vi "DROPBEAR_Model_Updating_FFT.vi"(8 "error in (no error)":errorcluster, 11 "DROPBEAR_Model_Updating in":refnum<class "DROPBEAR_Model_Updating.lvclass">=refnum) -> (0 "error out":errorcluster, 3 "DROPBEAR_Model_Updating out":refnum<class "DROPBEAR_Model_Updating.lvclass">, 4 "looping":bool=TRUE)   [LabVIEW 2021, in "DROPBEAR_Model_Updating.lvclass"]
uses:
  DROPBEAR_Model_Updating.lvclass
  MOCKBEAR/MOCKBEAR.lvclass
  FEA_Model/FEA_Model.lvclass
  Kalman_Filter/Kalman_Filter.lvclass
  Data_Array/Data_Array.lvclass
  Moving_Statistic/Moving_Statistic.lvclass
  Online_Statistic/Online_Statistic.lvclass
  <vilib>/Analysis/4window.llb/Hanning Window (DBL).vi
  <vilib>/Analysis/5stat.llb/RMS (DBL).vi
  <vilib>/Analysis/2dsp.llb/Real FFT.vi
  <vilib>/Analysis/4window.llb/AllCosWindow (DBL).vi
  <vilib>/Analysis/NI_AALPro.lvlib
panel:
  in  "Bound to 1st Frequency":bool=TRUE
  in  "Frequency Method":T1(ring)=enum."FFT"
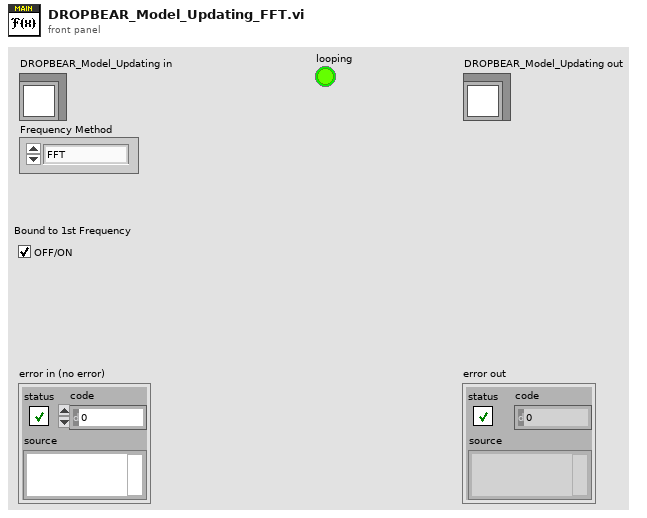
[diagram p1: front panel]
types:
  T1 = enum16{"Bandpass FFT", "Tone", "FFT", "Custom Filter"}
  T2 = cluster{"Time Cycle Start":u32, "Time Data Acquire":u32, "Time FFT":u32, "Time KF FFT":u32, "Time Sample":u32, "Time FEA":u32, "Time KF FEA":u32, "Time Cycle End":u32}
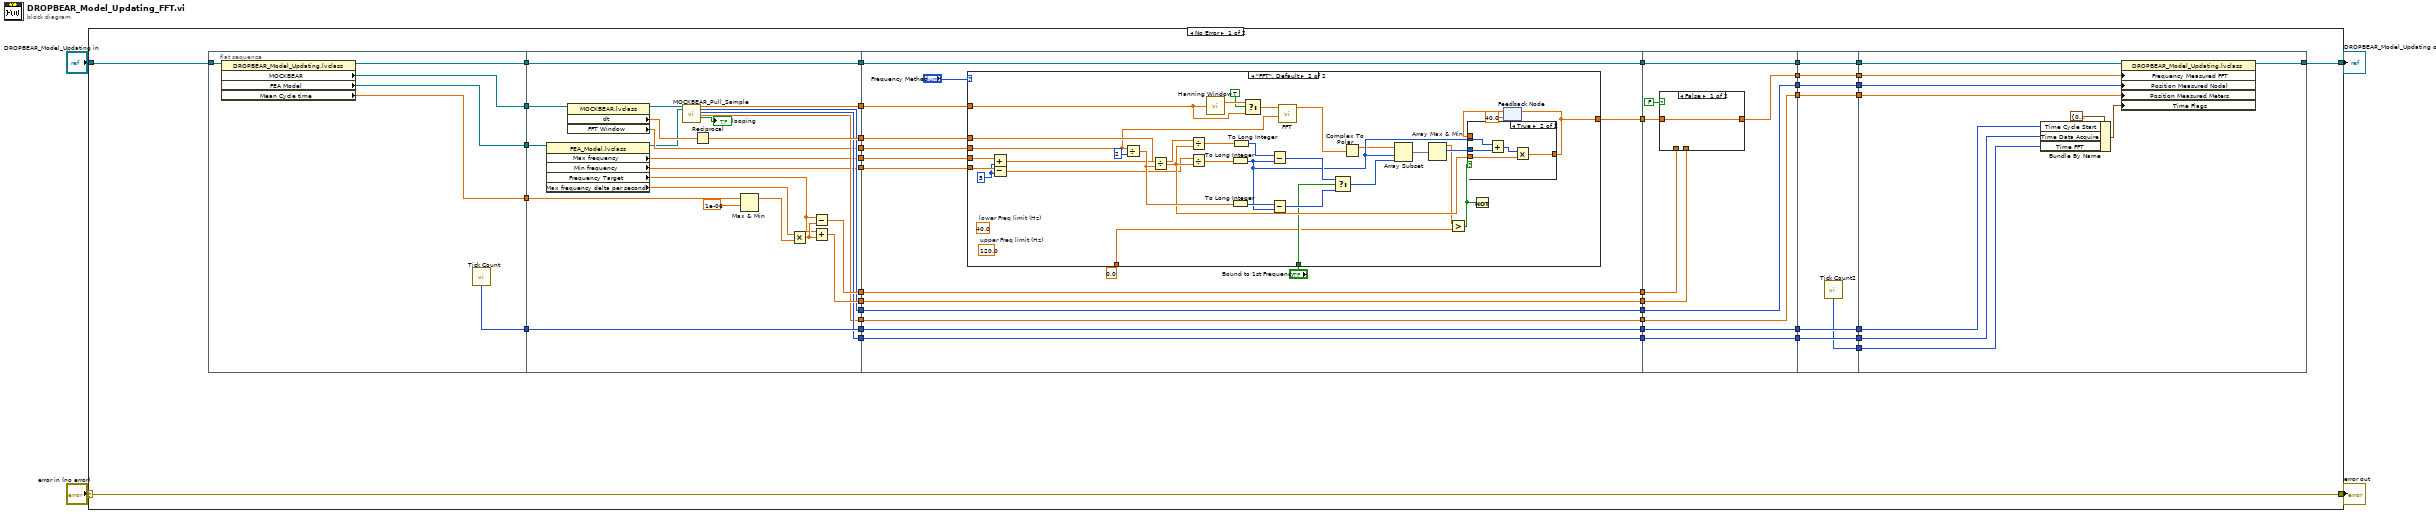
[diagram p0: block diagram]
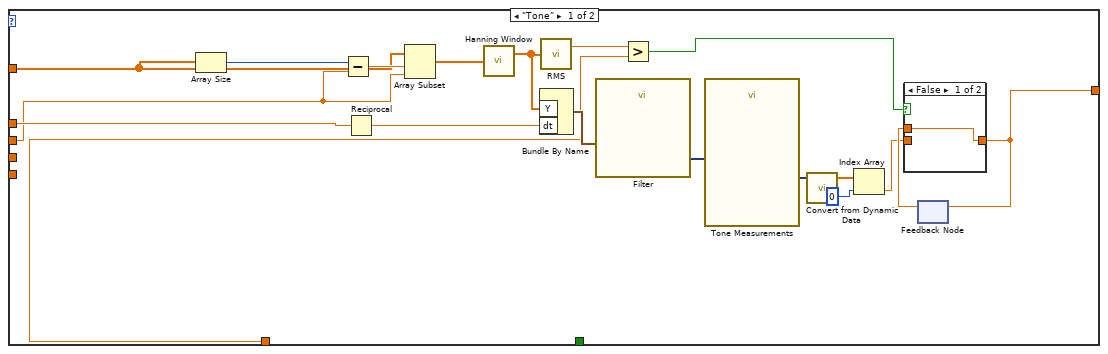
[diagram p2: hidden frame]
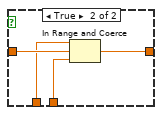
[diagram p5: hidden frame]
diagram:
  n1 = case shown="No Error" "error in (no error)" {
    selector: "error in (no error)" -> [w45 w185]
    tunnel: [w45 w185] -> w3
    tunnel: [w30 w184] -> w1
    tunnel: "DROPBEAR_Model_Updating in" -> [w19 w184]
    frame No Error {
      n2 = flat-sequence {
        tunnel: w19 -> [w50]
        tunnel: [w46] -> w44
        tunnel: [w48] -> w43
        tunnel: [w51] -> w26
        tunnel: [w49] -> w18
        tunnel: [w47] -> w9
        tunnel: w44 -> [w58]
        tunnel: w43 -> [w61]
        tunnel: [w72] -> w42
        tunnel: [w57] -> w41
        tunnel: [w56] -> w40
        tunnel: [w71] -> w39
        tunnel: [w59] -> w38
        tunnel: [w70] -> w37
        tunnel: [w69] -> w36
        tunnel: w26 -> [w68]
        tunnel: [w68] -> w25
        tunnel: [w67] -> w24
        tunnel: w18 -> [w66]
        tunnel: [w63] -> w17
        tunnel: [w62] -> w16
        tunnel: w9 -> [w52]
        tunnel: [w52] -> w8
        tunnel: w42 -> [w88]
        tunnel: w41 -> [w87]
        tunnel: w40 -> [w86]
        tunnel: w39 -> [w89]
        tunnel: w38 -> [w84]
        tunnel: w37 -> [w91]
        tunnel: w36 -> [w90]
        tunnel: [w91] -> w35
        tunnel: [w90] -> w34
        tunnel: [w83] -> w33
        tunnel: [w80] -> w28
        tunnel: w25 -> [w80]
        tunnel: w24 -> [w79]
        tunnel: [w79] -> w21
        tunnel: w17 -> [w78]
        tunnel: w16 -> [w77]
        tunnel: [w78] -> w15
        tunnel: [w77] -> w14
        tunnel: w8 -> [w76]
        tunnel: [w76] -> w7
        tunnel: w35 -> [w159]
        tunnel: w34 -> [w160]
        tunnel: w33 -> [w161]
        tunnel: [w158] -> w32
        tunnel: w28 -> [w156]
        tunnel: [w156] -> w27
        tunnel: [w155] -> w23
        tunnel: w21 -> [w155]
        tunnel: w15 -> [w154]
        tunnel: w14 -> [w153]
        tunnel: [w154] -> w12
        tunnel: [w153] -> w11
        tunnel: w7 -> [w152]
        tunnel: [w152] -> w6
        tunnel: w32 -> [w173]
        tunnel: [w173] -> w31
        tunnel: [w172] -> w29
        tunnel: w27 -> [w172]
        tunnel: w23 -> [w171]
        tunnel: [w171] -> w22
        tunnel: [w170] -> w20
        tunnel: [w169] -> w13
        tunnel: w12 -> [w169]
        tunnel: w11 -> [w168]
        tunnel: [w168] -> w10
        tunnel: w6 -> [w167]
        tunnel: [w167] -> w5
        tunnel: w31 -> [w183]
        tunnel: [w175] -> w30
        tunnel: w29 -> [w178]
        tunnel: w22 -> [w177]
        tunnel: w20 -> [w176]
        tunnel: w13 -> [w182]
        tunnel: w10 -> [w181]
        tunnel: w5 -> [w174]
        frame #0 {
          n3 = property class="DROPBEAR_Model_Updating.lvclass"(reference=w50) -> (reference out=w47:refnum<class "DROPBEAR_Model_Updating.lvclass">, "MOCKBEAR"=w49:refnum<class "MOCKBEAR.lvclass">, "FEA Model"=w46:refnum<class "FEA_Model.lvclass">, "Mean Cycle time"=w48:dbl)  [unwired: 1 in, 1 out]
          n4 = call "Tick Count"() -> ("Tick Count(uSec)"=w51:u32)
        }
        frame #1 {
          n5 = property class="FEA_Model.lvclass"(reference=w58) -> (reference out=w53:refnum<class "FEA_Model.lvclass">, "Max frequency"=w57:dbl, "Min frequency"=w56:dbl, "Frequency Target"=w55:dbl, "Max frequency delta per second"=w54:dbl)  [unwired: 1 in, 1 out]
          n6 = property class="MOCKBEAR.lvclass"(reference=w66) -> (reference out=w64:refnum<class "MOCKBEAR.lvclass">, "dt"=w65:dbl, "FFT Window"=w59:dbl)  [unwired: 1 in, 1 out]
          n7 = call "MOCKBEAR_Pull_Sample.vi"("MOCKBEAR in"=w64, "FEA Model"=w53) -> ("Accelerometer sample"=w71:dbl[], "Last pin pos node"=w63:i32, "Sample Time"=w67:u32, "Last pin pos meter"=w62:dbl, "looping"=→"looping":bool)  [unwired: 12 in, 1 out]
          n8 = Reciprocal(x=w65) -> (1/x=w72:dbl)
          n9 = Max & Min(x=w61, y=1e-06) -> (max(x,y)=w75:dbl)  [unwired: 1 out]
          n10 = Multiply(x=w54, y=w75) -> (x*y=w74:dbl)
          n11 = Subtract(x=w55, y=w74) -> (x-y=w70:dbl)
          n12 = Add(x=w55, y=w74) -> (x+y=w69:dbl)
        }
        frame #2 {
          n13 = case shown="\"FFT\", Default" "Frequency Method" {
            tunnel: [w98 w121] -> w83
            tunnel: w89 -> [w102 w115]
            tunnel: "Bound to 1st Frequency" -> [_ w133]
            tunnel: w88 -> [w94 w125]
            tunnel: w87 -> [_ w122]
            tunnel: w86 -> [_ w118]
            tunnel: 0.0 -> [w92 w123]
            tunnel: w84 -> [w93 w124]
            frame "Tone" {
              n14 = Array Size(array=w102) -> (size(s)=w110:i32)
              n15 = Subtract(x=w110, y=w93) -> (x-y=w109:dbl)
              n16 = Reciprocal(x=w94) -> (1/x=w95:dbl)
              n17 = Array Subset(array=w102, index=w109, length=w93) -> (w103:dbl[])
              n18 = call-poly <vilib>:"Hanning Window.vi"("X"=w103) -> ("Windowed X"=w100:dbl[])  [unwired: 1 out]
              n19 = Bundle By Name("Y"=w100, "dt"=w95) -> (w104:waveform(dbl))  [unwired: 1 in]
              n20 = call-poly <vilib>:"RMS.vi"("X"=w100) -> ("rms value"=w96:dbl)  [unwired: 1 out]
              n21 = call "Filter"("Signal"=w104) -> ("Filtered Signal"=w105:dynamicdata)  [unwired: 9 in, 1 out]
              n22 = Greater?(x=w96, y=w92) -> (0:w97:bool)
              n23 = call "Tone Measurements"("Signals"=w105) -> ("Frequency"=w106:dynamicdata)  [unwired: 9 in, 1 out]
              n24 = call "Convert from Dynamic Data"("Dynamic Data Type"=w106) -> ("Array"=w107:dbl[])  [unwired: 3 in]
              n25 = Index Array(array=w107, index=0) -> (element=w99:dbl)
              n26 = feedback #1() -> (w101:dbl)  [unwired: 1 in]
              n27 = case shown="False" w97 {
                tunnel: [w111 w112] -> w98
                tunnel: w101 -> [w111 _]
                tunnel: w99 -> [_ w112]
                frame False {
                }
                frame True {
                }
              }
              n28 = feedback-in #1(w98) -> ()
            }
            frame "FFT", Default {
              w113 = 5 ("y")
              (unwired) 120.0  # upper Freq limit (Hz)
              (unwired) 40.0  # lower Freq limit (Hz)
              n29 = Add(x=w122, y=w113) -> (x+y=w127:dbl)
              n30 = Subtract(x=w118, y=w113) -> (x-y=w128:dbl)
              n31 = Divide(x=w124, y=2) -> (x/y=w141:dbl)
              n32 = Divide(x=w125, y=w141) -> (x/y=w139:dbl)
              n33 = Divide(x=w127, y=w139) -> (x/y=w138:dbl)
              n34 = Divide(x=w128, y=w139) -> (x/y=w144:dbl)
              n35 = call-poly <vilib>:"Hanning Window.vi"("X"=w115) -> ("Windowed X"=w117:dbl[])  [unwired: 1 out]
              n36 = To Long Integer(number=w144) -> (32bit integer=w129:i32)
              n37 = To Long Integer(number=w141) -> (32bit integer=w142:i32)
              n38 = To Long Integer(number=w138) -> (32bit integer=w137:i32)
              n39 = Select(t=w117, s=TRUE, f=w115) -> (s? t:f=w114:dbl[])
              n40 = Subtract(x=w137, y=w129) -> (x-y=w135:i32)
              n41 = Subtract(x=w142, y=w129) -> (x-y=w134:i32)
              n42 = call-poly <vilib>:"FFT.vi"("FFT size"=w124, "X"=w114) -> ("FFT {X}"=w132:cdb[])  [unwired: 8 in, 1 out]
              n43 = Select(t=w135, s=w133, f=w134) -> (s? t:f=w136:i32)
              n44 = Complex To Polar(r * e^(i*theta)=w132) -> (r=w120:dbl[])  [unwired: 1 out]
              n45 = Array Subset(array=w120, index=w129, length=w136) -> (w119:dbl[])
              n46 = Array Max & Min(array=w119) -> (max value=w126:dbl, max index (indices)=w143:i32)  [unwired: 2 out]
              n47 = Greater?(x=w126, y=w123) -> (0:w140:bool)
              n48 = Not(x=w140) -> ()  [unwired: 1 out]
              n49 = feedback #2(40.0) -> (w131:dbl)
              n50 = case shown="True" w140 {
                tunnel: w143 -> [_ w148]
                tunnel: w129 -> [_ w149]
                tunnel: w139 -> [_ w150]
                tunnel: [w146 w147] -> w121
                tunnel: w131 -> [w146 _]
                frame False {
                }
                frame True {
                  n51 = Add(x=w149, y=w148) -> (x+y=w151:i32)
                  n52 = Multiply(x=w151, y=w150) -> (x*y=w147:dbl)
                }
              }
              n53 = feedback-in #2(w121) -> ()
            }
          }
        }
        frame #3 {
          n54 = case shown="False" FALSE {
            tunnel: w161 -> [w162 w166]
            tunnel: [w162 w165] -> w158
            tunnel: w160 -> [_ w163]
            tunnel: w159 -> [_ w164]
            frame False {
            }
            frame True {
              n55 = In Range and Coerce(upper limit=w164, x=w166, lower limit=w163) -> (coerced(x)=w165:dbl)  [unwired: 1 out]
            }
          }
        }
        frame #4 {
          n56 = call "Tick Count2"() -> ("Tick Count(uSec)"=w170:u32)
        }
        frame #5 {
          n57 = Bundle By Name(cluster=T2 {"Time Cycle Start"=0, "Time Data Acquire"=0, "Time FFT"=0, "Time KF FFT"=0, "Time Sample"=0, "Time FEA"=0, "Time KF FEA"=0, "Time Cycle End"=0} ("Time Flags"), "Time Cycle Start"=w178, "Time Data Acquire"=w177, "Time FFT"=w176) -> (w179:T2)
          n58 = property class="DROPBEAR_Model_Updating.lvclass"(reference=w174, "Frequency Measured FFT"=w183, "Position Measured Nodal"=w182, "Position Measured Meters"=w181, "Time Flags"=w179) -> (reference out=w175:refnum<class "DROPBEAR_Model_Updating.lvclass">)  [unwired: 1 in, 1 out]
        }
      }
    }
    frame Error {
    }
  }
  "error out" <- w3
  "DROPBEAR_Model_Updating out" <- w1
